vi "HXG2compFGV.vi"(7 "CompFGV":T1, 8 "error in (no error)":errorcluster, 11 "RUN?":bool) -> (0 "error out":errorcluster, 3 "RUN?":bool)   [LabVIEW 2012]
uses:
  HXG2comp.ctl
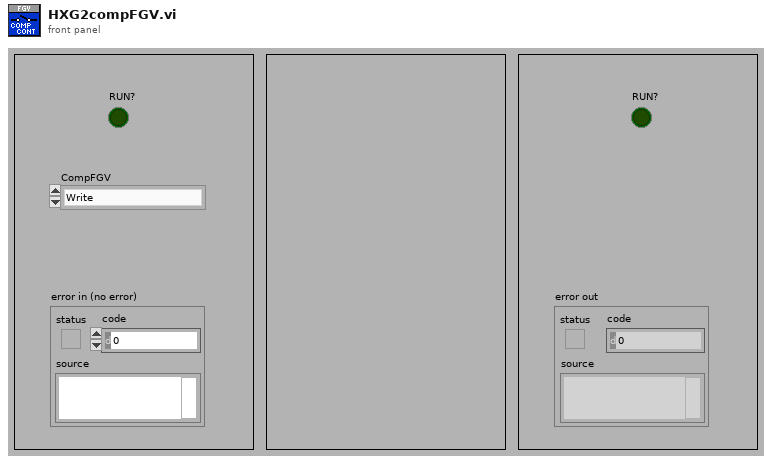
[diagram p1: front panel]
types:
  T1 = typedef "HXG2comp.ctl" = enum16{"Write", "Pass"}
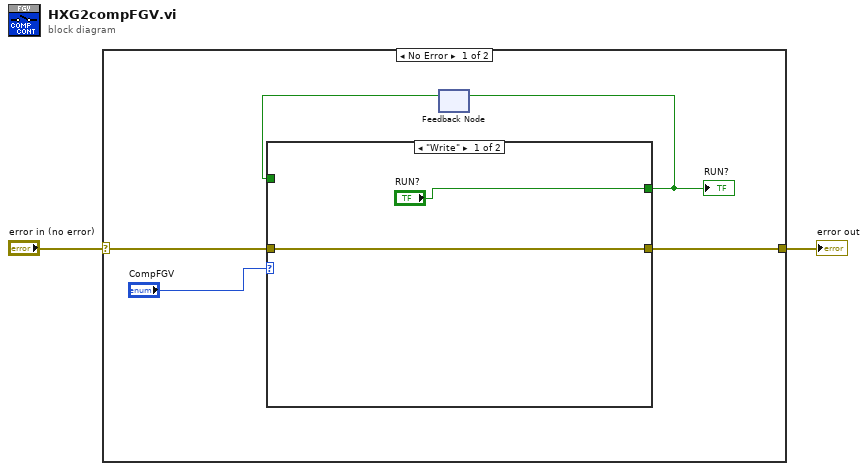
[diagram p0: block diagram]
diagram:
  n1 = case shown="No Error" "error in (no error)" {
    selector: "error in (no error)" -> [w7 w12]
    tunnel: [w6 w12] -> w1
    frame No Error {
      n2 = feedback #1() -> (w4:bool)  [unwired: 1 in]
      n3 = case shown="\"Write\"" "CompFGV" {
        tunnel: w7 -> [w8 w10]
        tunnel: [w8 w10] -> w6
        tunnel: ["RUN?" w11] -> w5
        tunnel: w4 -> [_ w11]
        frame "Write" {
        }
        frame "Pass" {
        }
      }
      "RUN?" <- w5
      n4 = feedback-in #1(w5) -> ()
    }
    frame Error {
    }
  }
  "error out" <- w1
